vi "Parse NT Boolean.vi"(11 "TCP Network Connection in":refnum<k5>) -> (2 "Boolean":bool, 3 "TCP Network Connection out":refnum<k5>)   [LabVIEW 2017]
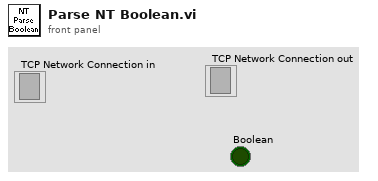
[diagram p1: front panel]
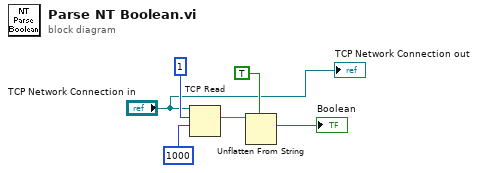
[diagram p0: block diagram]
diagram:
  n1 = TCP Read(connection ID="TCP Network Connection in", bytes to read=1 ("timeout ms (25000)"), 9:1000 ("timeout ms (25000)")) -> (data out=w4:string)  [unwired: 2 in, 2 out]
  n2 = Unflatten From String(type=TRUE, binary string=w4) -> (value=→"Boolean":bool)  [unwired: 3 in, 2 out]
  "TCP Network Connection out" <- "TCP Network Connection in"
